vi "GetOutputDir.vi"(8 "error in (no error)":errorcluster, 11 "SaveForPrevious in":refnum<class "SaveForPrevious.lvclass">) -> (0 "error out":errorcluster, 2 "TempDir":string, 3 "SaveForPrevious out":refnum<class "SaveForPrevious.lvclass">)   [LabVIEW 2014, in "SaveForPrevious.lvclass"]
doc: "Gets a temporary path where the files will be downgraded."
uses:
  SaveForPrevious.lvclass
  SaveForPrevious.lvclass/SaveForPrevious.ctl
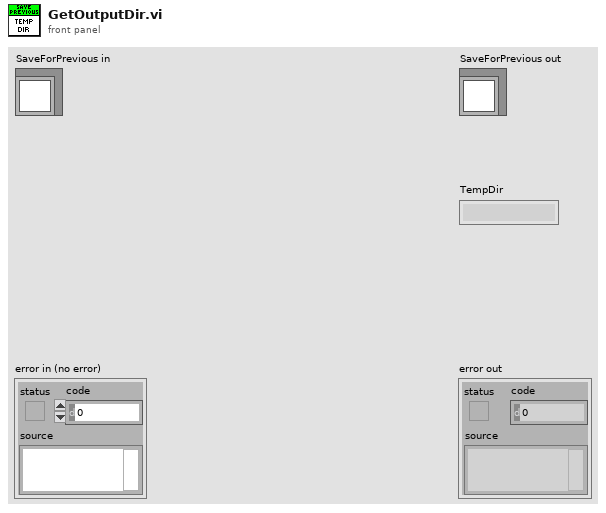
[diagram p1: front panel]
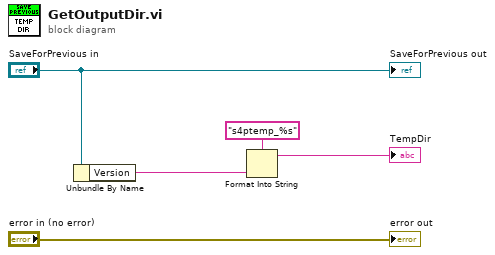
[diagram p0: block diagram]
diagram:
  n1 = Unbundle By Name("SaveForPrevious in") -> ("Version"=w2:string)
  n2 = Format Into String(format string="s4ptemp_%s" ("TempDir"), w2) -> (resulting string=→"TempDir":string)  [unwired: 2 in, 1 out]
  "error out" <- "error in (no error)"
  "SaveForPrevious out" <- "SaveForPrevious in"
